vi "日期时间记录-秒.vi"(11 "日期时间记录":T1) -> (3 "秒":dbl)   [LabVIEW 2013]
uses:
  <vilib>/Utility/miscctls.llb/LVDateTimeRec.ctl
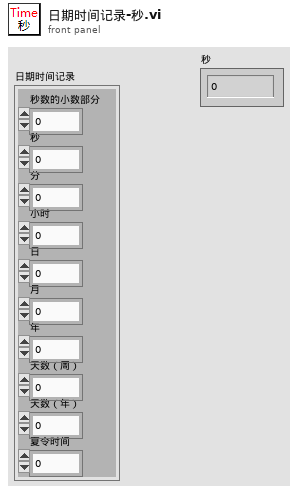
[diagram p1: front panel]
types:
  T1 = typedef "LVDateTimeRec.ctl" = cluster{"fractional second":dbl, "second":i32, "minute":i32, "hour":i32, "day of month":i32, "month":i32, "year":i32, "day of week":i32, "day of year":i32, "DST":i32}
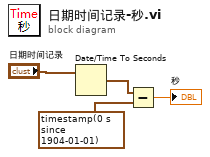
[diagram p0: block diagram]
diagram:
  n1 = Date/Time To Seconds(2:"日期时间记录") -> (0:w3:timestamp)  [unwired: 1 in]
  n2 = Subtract(x=w3, y=timestamp(0 s since 1904-01-01)) -> (x-y=→"秒":dbl)
